vi "NewtonsPSM_Meas_Harm_Series.vi"(0 "VISA session":refnum<visa-resource-name>, 9 "Scale (%)":bool, 11 "error in (no error)":errorcluster) -> (4 "dup VISA session":refnum<visa-resource-name>, 6 "Read Strings":string, 8 "Ch 1 Harmonic Graph":dbl[](graph), 10 "Ch 2 Harmonic Graph":dbl[](graph), 15 "error out":errorcluster)   [LabVIEW 2025, in "NewtonsPSM1735.lvlib"]
doc: "This VI reads the Harmonics series table from the PPA2530"
uses:
  NewtonsPSM1735.lvlib
panel:
  out "Ch 2 Phase Graph":dbl[](graph)
  out "Ch 1 Phase Graph":dbl[](graph)
  # "absolute"
  # "%"
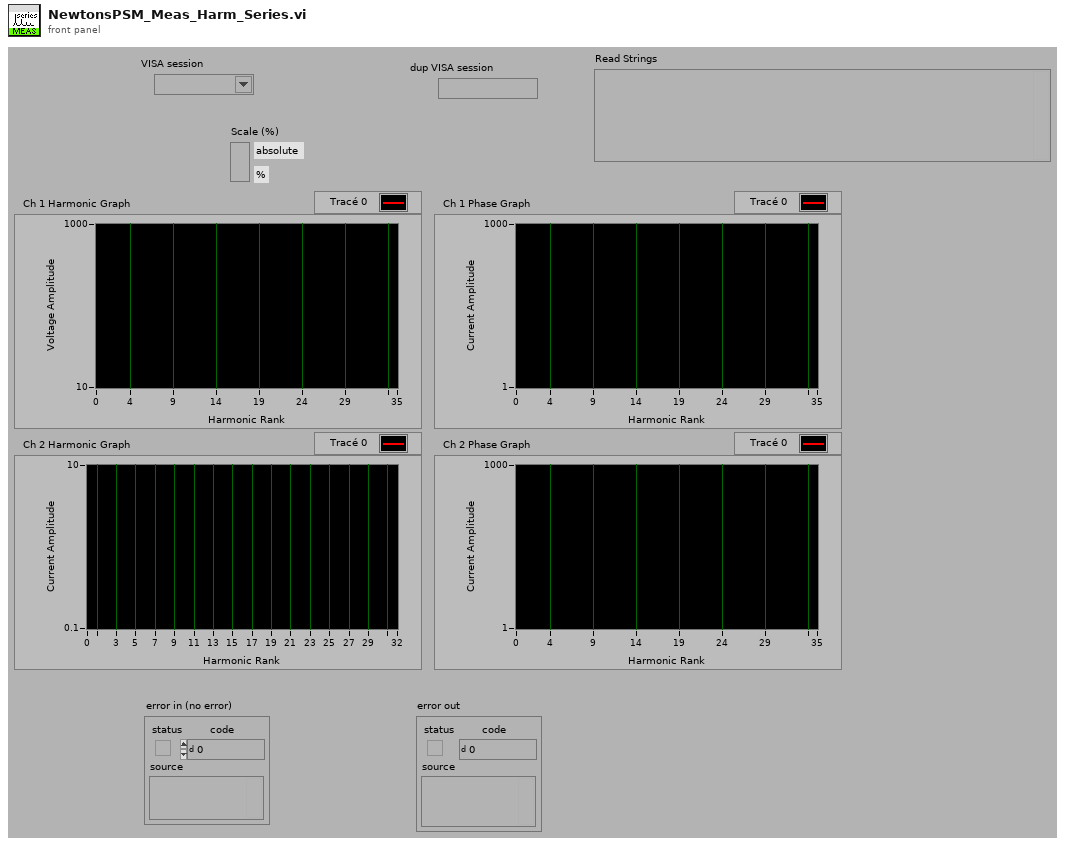
[diagram p1: front panel]
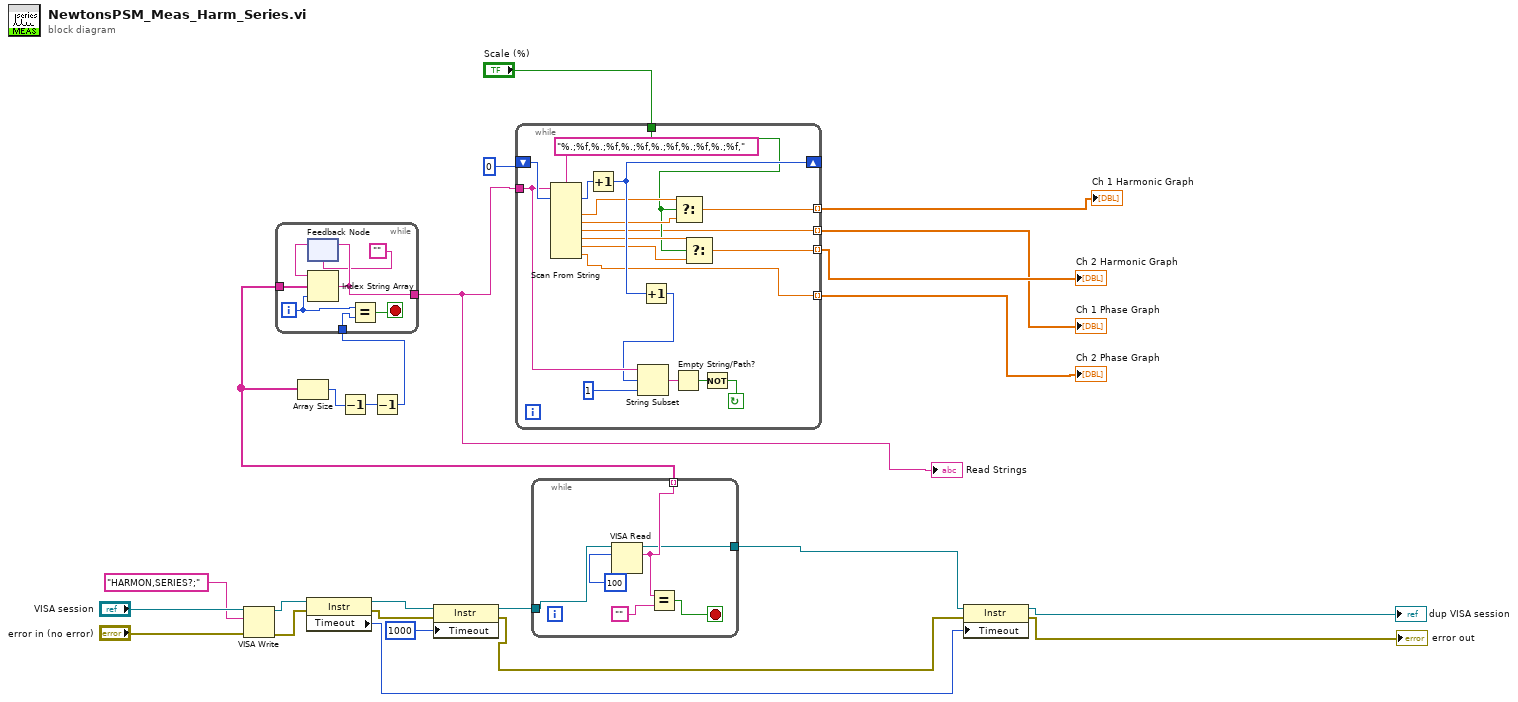
[diagram p0: block diagram]
diagram:
  n1 = VISA Write(VISA resource name="VISA session", write buffer="HARMON,SERIES?;", error in (no error)="error in (no error)") -> (VISA resource name out=w22:refnum<visa-resource-name>, error out=w21:errorcluster)  [unwired: 1 out]
  n2 = property class="Instr"(reference=w22, error in=w21) -> (reference out=w16:refnum<visa-resource-name>, error out=w17:errorcluster, "Timeout"=w18:u32)
  n3 = property class="Instr"(reference=w16, error in=w17, "Timeout"=u32 1000 ("General Settings:Timeout Value")) -> (reference out=w14:refnum<visa-resource-name>, error out=w13:errorcluster)
  n4 = while {
    tunnel: w14 -> [w30]
    tunnel: [w27] -> w8 mode=indexing
    tunnel: [w26] -> w12
    stop <- w29 stop-if-true
    n5 = VISA Read(VISA resource name=w30, byte count=u32 100 ("ÊÞ²Ä¶³ÝÄi0j")) -> (VISA resource name out=w26:refnum<visa-resource-name>, read buffer=w27:string)  [unwired: 1 in, 2 out]
    n6 = Equal?(x=w27, y="") -> (x = y?=w29:bool)
  }
  n7 = Array Size(array=w8) -> (size(s)=w11:i32)
  n8 = Decrement(x=w11) -> (x-1=w10:i32)
  n9 = Decrement(x=w10) -> (x-1=w9:i32)
  n10 = while {
    tunnel: w8 -> [w38]
    tunnel: [w36] -> w2
    tunnel: w9 -> [w34]
    i -> [w35]
    stop <- w37 stop-if-true
    n11 = feedback #1("") -> (w33:string)
    n12 = Index String Array(1:w35, 2:w38, 3:w33) -> (0:w36:string)
    n13 = feedback-in #1(w36) -> ()
    n14 = Equal?(x=w35, y=w34) -> (x = y?=w37:bool)
  }
  "Read Strings" <- w2
  n15 = while {
    shift-left: u32 0 -> [w51]
    shift-right: [w49] -> _
    tunnel: w2 -> [w50]
    tunnel: "Scale (%)" -> [w43]
    tunnel: [w42] -> w6 mode=indexing
    tunnel: [w41] -> w5 mode=indexing
    tunnel: [w40] -> w4 mode=indexing
    tunnel: [w39] -> w3 mode=indexing
    stop <- w54 continue-if-true
    n16 = Scan From String(format string="%.;%f,%.;%f,%.;%f,%.;%f,%.;%f,%.;%f,", input string=w50, initial scan location=w51) -> (offset past scan=w52:u32, output 1=w47:dbl, output 2=w46:dbl, output 3=w40:dbl, output 4=w45:dbl, output 5=w44:dbl, output 6=w39:dbl)  [unwired: 1 in, 8 out]
    n17 = Increment(x=w52) -> (x+1=w49:u32)
    n18 = Increment(x=w49) -> (x+1=w48:u32)
    n19 = String Subset(string=w50, offset (0)=w48, length (rest)=1) -> (substring=w56:string)
    n20 = Empty String/Path?(string/path=w56) -> (empty?=w55:bool)
    n21 = Select(t=w47, s=w43, f=w46) -> (s? t:f=w42:dbl)
    n22 = Select(t=w45, s=w43, f=w44) -> (s? t:f=w41:dbl)
    n23 = Not(x=w55) -> (.not. x?=w54:bool)
  }
  "Ch 1 Harmonic Graph" <- w6
  "Ch 2 Harmonic Graph" <- w5
  "Ch 1 Phase Graph" <- w4
  "Ch 2 Phase Graph" <- w3
  n24 = property class="Instr"(reference=w12, error in=w13, "Timeout"=w18) -> (reference out=→"dup VISA session":refnum<visa-resource-name>, error out=→"error out":errorcluster)
